vi "Sweep control - Copy.vi"(0 "Scan control":cluster{"Priority":u16, "Scan name":u16}[](array[cluster])=[{"Priority"=0, "Scan name"=1}, {"Priority"=3, "Scan name"=0}, {"Priority"=2, "Scan name"=0}, {"Priority"=1, "Scan name"=6}] {"Scan name" items=["OFF", "Vsg1", "Vsg2", "Vsgw", "Vbg", "Field", "Temp"]; "Priority" items=["Priority 0", "Priority 1", "Priority 2", "Priority 3", "Priority 4", "Priority 5"]}, 1 "Scan parameters":T2(array[cluster])=[{"DAQ Channel"=1, "Label"="\nappliedVsg=", "Scaled low"=-0.1, "Scaled high"=0.1, "Start"=-0.1, "End"=0.1, "Step"=0.0002, "Scale?"=FALSE}, {"DAQ Channel"=2, "Label"="\nappliedVsg2=", "Scaled low"=-0.175, "Scaled high"=0.775, "Start"=-0.05, "End"=0.25, "Step"=0.0003, "Scale?"=FALSE}, {"DAQ Channel"=3, "Label"="\nappliedVbg=", "Scaled low"=-0.11, "Scaled high"=0.31, "Start"=-10.0, "End"=4.0, "Step"=0.005, "Scale?"=FALSE}, {"DAQ Channel"=3, "Label"="\nAppliedTemp=", "Scaled low"=-0.060000000000000005, "Scaled high"=0.14, "Start"=0.05, "End"=0.05, "Step"=0.001, "Scale?"=FALSE}] {"Step" format="%#_6f"; "End" format="%#_6f"; "Start" format="%#_6f"; "Scaled high" format="%#_6p"; "Scaled low" format="%#_6p"}, 2 "OSC Configuration":T1(array[cluster])=[{"Signal Type"=enum."Sawtooth Wave", "DC"=0.00035, "Amplitude"=0.003, "frequency"=0.4, "Phase"=180.0}, {"Signal Type"=enum."Sine Wave", "DC"=0.0, "Amplitude"=0.0, "frequency"=1.0, "Phase"=0.0}, {"Signal Type"=enum."Sine Wave", "DC"=0.0, "Amplitude"=0.0, "frequency"=1.0, "Phase"=0.0}, {"Signal Type"=enum."Sine Wave", "DC"=0.0, "Amplitude"=0.0, "frequency"=1.0, "Phase"=0.0}] {"frequency" format="%0.2p"; "Amplitude" format="%0.2p"; "DC" format="%.2p"}, 3 "Comments":string="SA02702H.201301106\n3mVac+350uVdc\nVbg= -0.3 V\nsweep Vsg from -0.1V to 0.075 V in step of 0.2mV\n", 4 "Experiment folder name":string="IV_Vsg sweep_Vbg-0.3V", 8 "Additional action (indexing priority)":u16[](array[ring])=[4, 1, 4, 4] items=["Clear DAQ Tasks", "Check Temperature", "Check Field Value", "Wait", "Do Nothing"]) -> ()   [LabVIEW 2013]
uses:
  lockin/branches/PPMS-demomode-JL/Lockin-4461_MultiChannel - IV 3.0 globals.vi
panel:
  in  "Number of IV curves":i32=1
  # "Instructions: \n1, you can put multiple scan names in one priority.\n2 OFF has to put in last priority"
  # "I wanted to check the temperature as well as the field (so the zero-field data isn't taken at higher temperatures) so I changed the post-action subvi slightly. In the 'check temperature' case, I made the stop condition that the temp is less than 70mK. By putting 'check temperature' with priority 1, i figure it'll set Vsg1&2 at 0, then wait for the temp to reach 70mK, before it starts sweeping prioity 0."
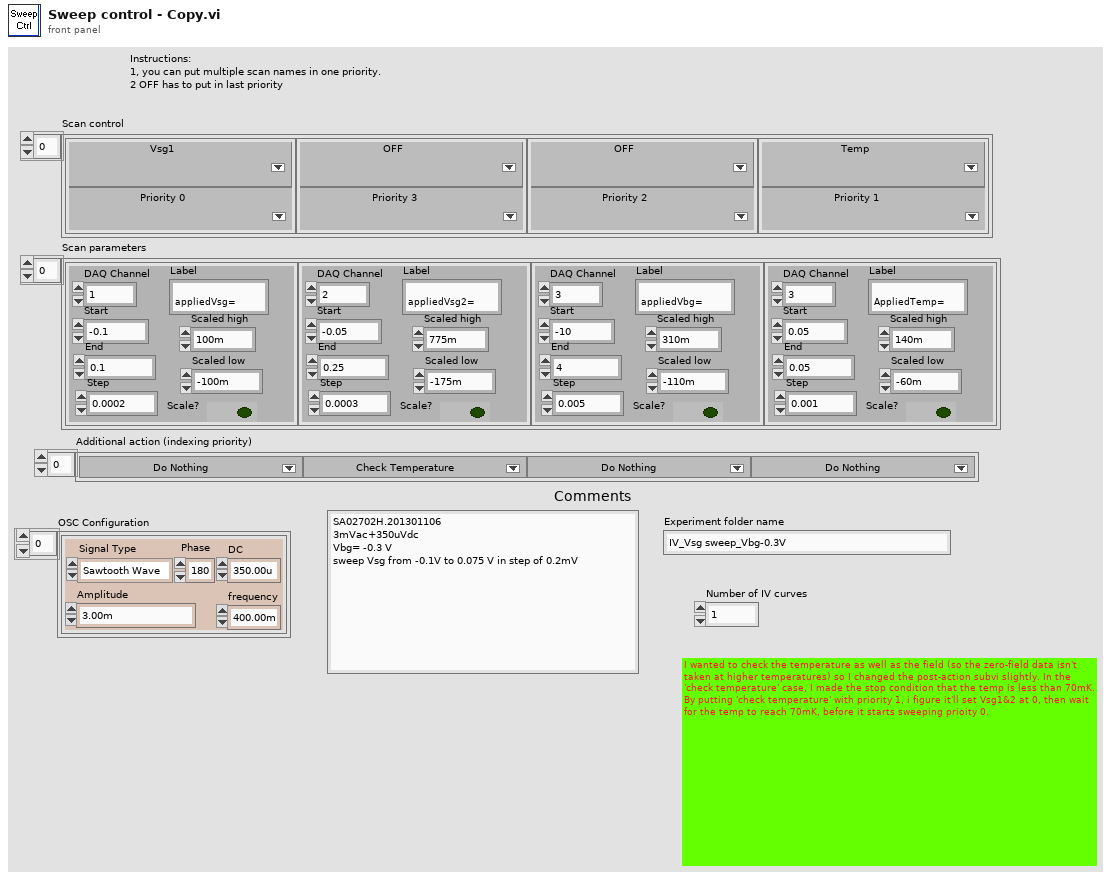
[diagram p1: front panel]
types:
  T1 = cluster{"Signal Type":enum16{"Sine Wave", "Triangle Wave", "Square Wave", "Sawtooth Wave"}, "DC":dbl, "Amplitude":dbl, "frequency":dbl, "Phase":dbl}[]
  T2 = cluster{"DAQ Channel":i32, "Label":string, "Scaled low":dbl, "Scaled high":dbl, "Start":dbl, "End":dbl, "Step":dbl, "Scale?":bool}[]
  T3 = cluster{cluster{"DAQ Channel":i32, "Label":string, "Scaled low":dbl, "Scaled high":dbl, "Start":dbl, "End":dbl, "Step":dbl, "Scale?":bool}[]}[]
  T4 = cluster{cluster{"Priority":u16, "Scan name":u16}[]}[]
  T5 = cluster{cluster{"DAQ Channel":i32, "Label":string, "Scaled low":dbl, "Scaled high":dbl, "Start":dbl, "End":dbl, "Step":dbl, "Scale?":bool}[]}
  T6 = cluster{cluster{"Priority":u16, "Scan name":u16}[]}
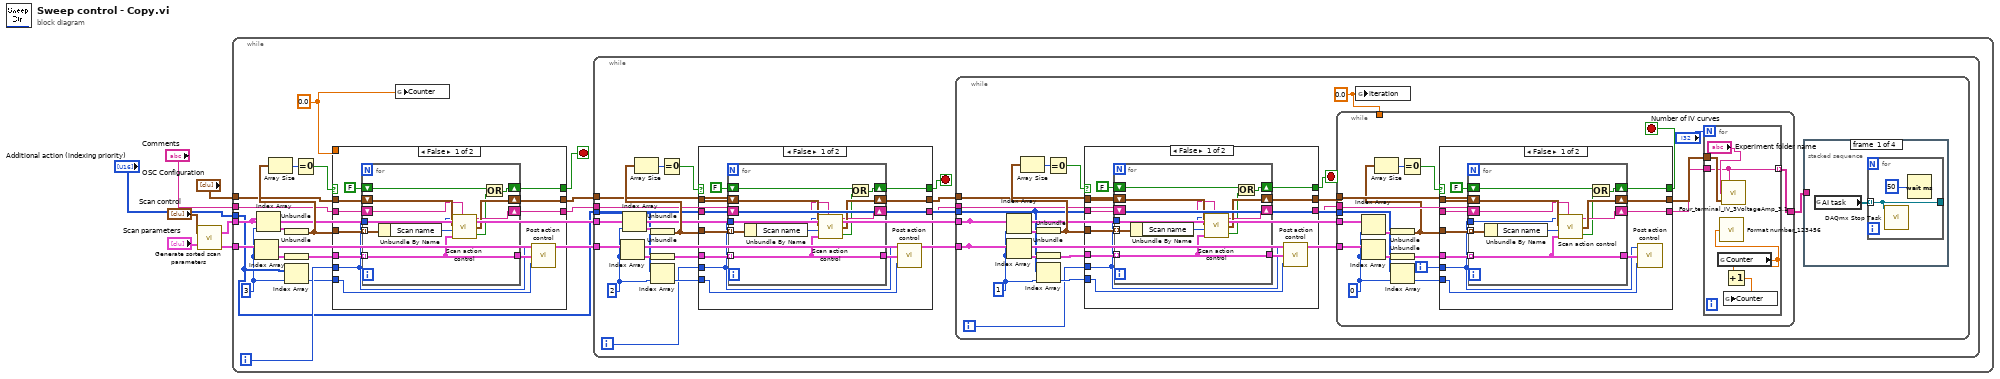
[diagram p0: block diagram]
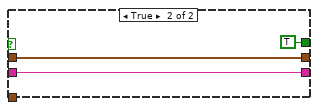
[diagram p2: hidden frame]
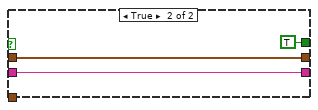
[diagram p3: hidden frame]
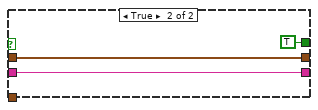
[diagram p4: hidden frame]
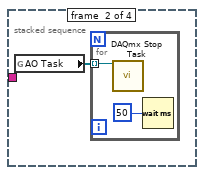
[diagram p5: hidden frame]
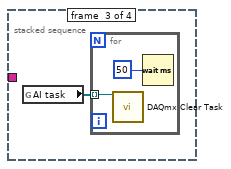
[diagram p6: hidden frame]
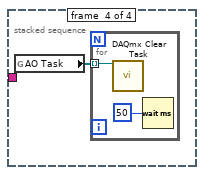
[diagram p7: hidden frame]
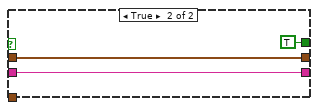
[diagram p8: hidden frame]
diagram:
  n1 = call "Generate sorted scan parameters.vi"("Scan parameters"="Scan parameters", "Scan control"="Scan control") -> ("Sorted scan parameters"=w3:T3, "Sorted scan control"=w2:T4)
  n2 = while {
    tunnel: "Comments" -> [w12]
    tunnel: "OSC Configuration" -> [w13]
    tunnel: w3 -> [w20]
    tunnel: w2 -> [w19]
    tunnel: "Additional action (indexing priority)" -> [w14]
    i -> [w16]
    stop <- w17 stop-if-true
    w8 = 0.0 ("IV count")
    w9 = 3
    n3 = Index Array(array=w20, index=w9) -> (element=w21:T5)
    n4 = Index Array(array=w19, index=w9) -> (element=w18:T6)
    n5 = Unbundle(w18) -> (w23:cluster{"Priority":u16, "Scan name":u16}[])
    n6 = Array Size(array=w23) -> (size(s)=w24:i32)
    n7 = Unbundle(w21) -> (w22:T2)
    n8 = Index Array(array=w14, index=w9) -> (element=w15:u16)
    n9 = Equal To 0?(x=w24) -> (x = 0?=w25:bool)
    n10 = case shown="False" w25 {
      tunnel: w22 -> [w36 _]
      tunnel: [w35 w49] -> w11
      tunnel: [w34 w48] -> w10
      tunnel: [w28 TRUE ("Stop?")] -> w17
      tunnel: w23 -> [w33 _]
      tunnel: w16 -> [w30 _]
      tunnel: w15 -> [w31 _]
      tunnel: w13 -> [w27 w49]
      tunnel: w12 -> [w26 w48]
      tunnel: w8 -> [_ _]
      frame False {
        n11 = for {
          tunnel: w33 -> [w47] mode=indexing
          tunnel: w36 -> [w40] mode=indexing
          tunnel: w30 -> [w41]
          shift-right: [w45] -> w35
          shift-left: w27 -> [w44]
          shift-right: [w43] -> w34
          shift-left: w26 -> [w42]
          tunnel: [w40] -> w32
          shift-right: [w37] -> w28
          shift-left: FALSE -> [w39]
          n12 = Unbundle By Name(w47) -> ("Scan name"=w46:u16)
          n13 = call "Scan action control.vi"("Index"=w41, "OSC Configuration"=w44, "Scan control"=w46, "Scan Parameters"=w40, "Comments"=w42) -> ("Comments out"=w43:string, "OSC Configuration out"=w45:T1, "Stop?"=w38:bool)
          n14 = Or(x=w39, y=w38) -> (x .or. y?=w37:bool)
        }
        n15 = call "Post action control.vi"("Action"=w31, "Scan Parameters"=w32, "Index"=w30) -> ()  [unwired: 1 out]
      }
      frame True {
      }
    }
    n16 = global write "Lockin-4461_MultiChannel - IV 3.0 globals.vi" "Counter"(w8) -> ()
    n17 = while {
      tunnel: w20 -> [w60]
      tunnel: w19 -> [w59]
      tunnel: w14 -> [w58]
      tunnel: w10 -> [w57]
      tunnel: w11 -> [w56]
      i -> [w55]
      stop <- w54 stop-if-true
      w51 = 2
      n18 = Index Array(array=w60, index=w51) -> (element=w66:T5)
      n19 = Index Array(array=w59, index=w51) -> (element=w67:T6)
      n20 = Unbundle(w67) -> (w64:cluster{"Priority":u16, "Scan name":u16}[])
      n21 = Array Size(array=w64) -> (size(s)=w62:i32)
      n22 = Unbundle(w66) -> (w65:T2)
      n23 = Index Array(array=w58, index=w51) -> (element=w63:u16)
      n24 = Equal To 0?(x=w62) -> (x = 0?=w61:bool)
      n25 = case shown="False" w61 {
        tunnel: w65 -> [w78 _]
        tunnel: w56 -> [w77 w92]
        tunnel: w57 -> [w76 w91]
        tunnel: [w75 w92] -> w53
        tunnel: [w74 w91] -> w52
        tunnel: [w68 TRUE ("Stop?")] -> w54
        tunnel: w64 -> [w73 _]
        tunnel: w55 -> [w70 _]
        tunnel: w63 -> [w71 _]
        frame False {
          n26 = for {
            tunnel: w73 -> [w89] mode=indexing
            tunnel: w78 -> [w82] mode=indexing
            tunnel: w70 -> [w83]
            shift-right: [w87] -> w75
            shift-left: w77 -> [w86]
            shift-right: [w85] -> w74
            shift-left: w76 -> [w84]
            tunnel: [w82] -> w72
            shift-right: [w79] -> w68
            shift-left: FALSE -> [w81]
            n27 = Unbundle By Name(w89) -> ("Scan name"=w88:u16)
            n28 = call "Scan action control.vi"("Index"=w83, "OSC Configuration"=w86, "Scan control"=w88, "Scan Parameters"=w82, "Comments"=w84) -> ("Comments out"=w85:string, "OSC Configuration out"=w87:T1, "Stop?"=w80:bool)
            n29 = Or(x=w81, y=w80) -> (x .or. y?=w79:bool)
          }
          n30 = call "Post action control.vi"("Action"=w71, "Scan Parameters"=w72, "Index"=w70) -> ()  [unwired: 1 out]
        }
        frame True {
        }
      }
      n31 = while {
        tunnel: w53 -> [w102]
        tunnel: w52 -> [w101]
        tunnel: w59 -> [w100]
        tunnel: w60 -> [w99]
        tunnel: w58 -> [w98]
        i -> [w93]
        stop <- w95 stop-if-true
        w94 = 1
        w111 = 0.0 ("iteration")
        n32 = Index Array(array=w100, index=w94) -> (element=w103:T6)
        n33 = Index Array(array=w99, index=w94) -> (element=w104:T5)
        n34 = Unbundle(w103) -> (w106:cluster{"Priority":u16, "Scan name":u16}[])
        n35 = Array Size(array=w106) -> (size(s)=w108:i32)
        n36 = Unbundle(w104) -> (w105:T2)
        n37 = Index Array(array=w98, index=w94) -> (element=w107:u16)
        n38 = Equal To 0?(x=w108) -> (x = 0?=w109:bool)
        n39 = case shown="False" w109 {
          tunnel: w105 -> [w122 _]
          tunnel: w102 -> [w121 w136]
          tunnel: w101 -> [w120 w135]
          tunnel: [w119 w136] -> w96
          tunnel: [w118 w135] -> w97
          tunnel: [w112 TRUE ("Stop?")] -> w95
          tunnel: w106 -> [w117 _]
          tunnel: w93 -> [w114 _]
          tunnel: w107 -> [w115 _]
          frame False {
            n40 = for {
              tunnel: w117 -> [w133] mode=indexing
              tunnel: w122 -> [w126] mode=indexing
              tunnel: w114 -> [w127]
              shift-right: [w131] -> w119
              shift-left: w121 -> [w130]
              shift-right: [w129] -> w118
              shift-left: w120 -> [w128]
              tunnel: [w126] -> w116
              shift-right: [w123] -> w112
              shift-left: FALSE -> [w125]
              n41 = Unbundle By Name(w133) -> ("Scan name"=w132:u16)
              n42 = call "Scan action control.vi"("Index"=w127, "OSC Configuration"=w130, "Scan control"=w132, "Scan Parameters"=w126, "Comments"=w128) -> ("Comments out"=w129:string, "OSC Configuration out"=w131:T1, "Stop?"=w124:bool)
              n43 = Or(x=w125, y=w124) -> (x .or. y?=w123:bool)
            }
            n44 = call "Post action control.vi"("Action"=w115, "Scan Parameters"=w116, "Index"=w114) -> ()  [unwired: 1 out]
          }
          frame True {
          }
        }
        n45 = while {
          tunnel: w100 -> [w166]
          tunnel: w99 -> [w165]
          tunnel: w96 -> [w161]
          tunnel: w97 -> [w160]
          tunnel: w98 -> [w154]
          tunnel: w111 -> [_]
          tunnel: [w150] -> w110
          i -> [w155]
          stop <- w157 stop-if-true
          w149 = 0
          n46 = Index Array(array=w166, index=w149) -> (element=w164:T6)
          n47 = Index Array(array=w165, index=w149) -> (element=w163:T5)
          n48 = Unbundle(w164) -> (w156:cluster{"Priority":u16, "Scan name":u16}[])
          n49 = Array Size(array=w156) -> (size(s)=w152:i32)
          n50 = Unbundle(w163) -> (w162:T2)
          n51 = Index Array(array=w154, index=w149) -> (element=w153:u16)
          n52 = Equal To 0?(x=w152) -> (x = 0?=w151:bool)
          n53 = case shown="False" w151 {
            tunnel: w162 -> [w178 _]
            tunnel: w161 -> [w177 w192]
            tunnel: w160 -> [w176 w191]
            tunnel: [w175 w192] -> w159
            tunnel: [w174 w191] -> w158
            tunnel: [w168 TRUE ("Stop?")] -> w157
            tunnel: w156 -> [w173 _]
            tunnel: w155 -> [w170 _]
            tunnel: w153 -> [w171 _]
            frame False {
              n54 = for {
                tunnel: w173 -> [w189] mode=indexing
                tunnel: w178 -> [w182] mode=indexing
                tunnel: w170 -> [w183]
                shift-right: [w187] -> w175
                shift-left: w177 -> [w186]
                shift-right: [w185] -> w174
                shift-left: w176 -> [w184]
                tunnel: [w182] -> w172
                shift-right: [w179] -> w168
                shift-left: FALSE -> [w181]
                n55 = Unbundle By Name(w189) -> ("Scan name"=w188:u16)
                n56 = call "Scan action control.vi"("Index"=w183, "OSC Configuration"=w186, "Scan control"=w188, "Scan Parameters"=w182, "Comments"=w184) -> ("Comments out"=w185:string, "OSC Configuration out"=w187:T1, "Stop?"=w180:bool)
                n57 = Or(x=w181, y=w180) -> (x .or. y?=w179:bool)
              }
              n58 = call "Post action control.vi"("Action"=w171, "Scan Parameters"=w172, "Index"=w170) -> ()  [unwired: 1 out]
            }
            frame True {
            }
          }
          n59 = for {
            N: "Number of IV curves" -> [_]
            tunnel: w159 -> [w194]
            tunnel: w158 -> [w193]
            tunnel: [w193] -> w150 mode=indexing
            n60 = global read "Lockin-4461_MultiChannel - IV 3.0 globals.vi" "Counter"() -> (w196:dbl)
            n61 = call <userlib>:"Format number_123456.vi"("number"=w196) -> ()  [unwired: 1 out]
            n62 = call "Four_terminal_IV_3VoltageAmp_3.1.vi"("Comments"=w193, "Experiment folder name"="Experiment folder name", "OSC Configuration"=w194) -> ()  [unwired: 1 in, 5 out]
            n63 = Increment(x=w196) -> (x+1=w197:dbl)
            n64 = global write "Lockin-4461_MultiChannel - IV 3.0 globals.vi" "Counter"(w197) -> ()
          }
        }
        n65 = global write "Lockin-4461_MultiChannel - IV 3.0 globals.vi" "iteration"(w111) -> ()
        n66 = stacked-sequence {
          tunnel: w110 -> [_ _ _ _]
          frame #0 {
            n67 = global read "Lockin-4461_MultiChannel - IV 3.0 globals.vi" "AI task"() -> (w137:refnum<k21>[])
            n68 = for {
              tunnel: w137 -> [w138] mode=indexing
              tunnel: [w138] -> _
              n69 = call <vilib>:"DAQmx Stop Task.vi"("task/channels in"=w138) -> ()  [unwired: 13 in, 2 out]
              n70 = Wait (ms)(milliseconds to wait=u32 50) -> ()  [unwired: 1 out]
            }
          }
          frame #1 {
            n71 = global read "Lockin-4461_MultiChannel - IV 3.0 globals.vi" "AO Task"() -> (w140:refnum<k21>[])
            n72 = for {
              tunnel: w140 -> [w142] mode=indexing
              n73 = call <vilib>:"DAQmx Stop Task.vi"("task/channels in"=w142) -> ()  [unwired: 13 in, 2 out]
              n74 = Wait (ms)(milliseconds to wait=u32 50) -> ()  [unwired: 1 out]
            }
          }
          frame #2 {
            n75 = global read "Lockin-4461_MultiChannel - IV 3.0 globals.vi" "AI task"() -> (w143:refnum<k21>[])
            n76 = for {
              tunnel: w143 -> [w145] mode=indexing
              n77 = call <vilib>:"DAQmx Clear Task.vi"("task in"=w145) -> ()  [unwired: 14 in, 1 out]
              n78 = Wait (ms)(milliseconds to wait=u32 50) -> ()  [unwired: 1 out]
            }
          }
          frame #3 {
            n79 = global read "Lockin-4461_MultiChannel - IV 3.0 globals.vi" "AO Task"() -> (w146:refnum<k21>[])
            n80 = for {
              tunnel: w146 -> [w148] mode=indexing
              n81 = call <vilib>:"DAQmx Clear Task.vi"("task in"=w148) -> ()  [unwired: 14 in, 1 out]
              n82 = Wait (ms)(milliseconds to wait=u32 50) -> ()  [unwired: 1 out]
            }
          }
        }
      }
    }
  }
